vi "選擇1P 2P.vi"() -> (2 "OK Button 4":bool, 3 "OK Button 3":bool)   [LabVIEW 2014]
panel:
  out "Boolean 3":bool
  out "Boolean 2":bool
  in  "OK Button 2":bool
  in  "OK Button":bool
  # "歡迎來到青蛙歷險記"
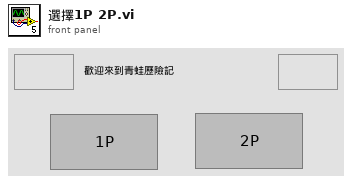
[diagram p1: front panel]
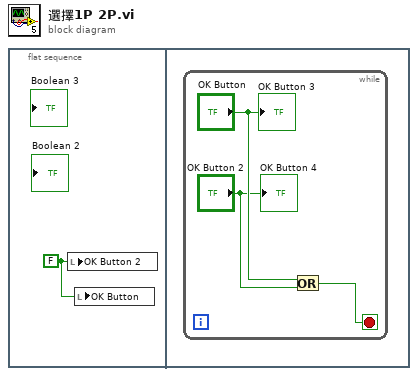
[diagram p0: block diagram]
diagram:
  n1 = flat-sequence {
    frame #0 {
      w1 = FALSE ("OK Button 2")
      n2 = local write "OK Button 2"(w1) -> ()
      n3 = local write "OK Button"(w1) -> ()
    }
    frame #1 {
      n4 = while {
        stop <- w2 stop-if-true
        n5 = Or(x="OK Button", y="OK Button 2") -> (x .or. y?=w2:bool)
        "OK Button 3" <- "OK Button"
        "OK Button 4" <- "OK Button 2"
      }
    }
  }
